vi "Assignment 1.vi"() -> ()   [LabVIEW 2023]
panel:
  out "Warning":string
  out "Kilometers":dbl
  in  "Miles":dbl
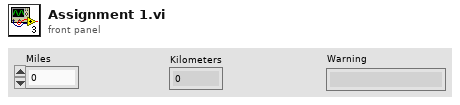
[diagram p1: front panel]
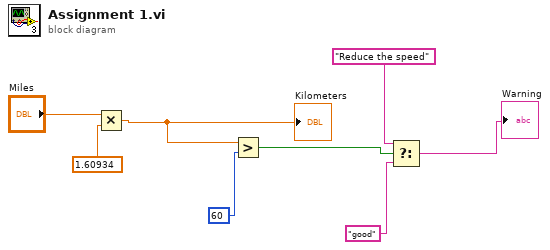
[diagram p0: block diagram]
diagram:
  n1 = Multiply(x="Miles", y=1.60934) -> (x*y=w1:dbl)
  "Kilometers" <- w1
  n2 = Greater?(x=w1, y=60) -> (0:w6:bool)
  n3 = Select(t="Reduce the speed", s=w6, f="good") -> (s? t:f=→"Warning":string)
